vi "ReversedEngineering GetRunTimeMenuTags.vi"(1 "StateMachineCaseSelector":path, 5 "error in":errorcluster) -> (16 "ItemTags":string[](array[string]), 19 "error out":errorcluster)   [LabVIEW 2014]
panel:
  out "data":string
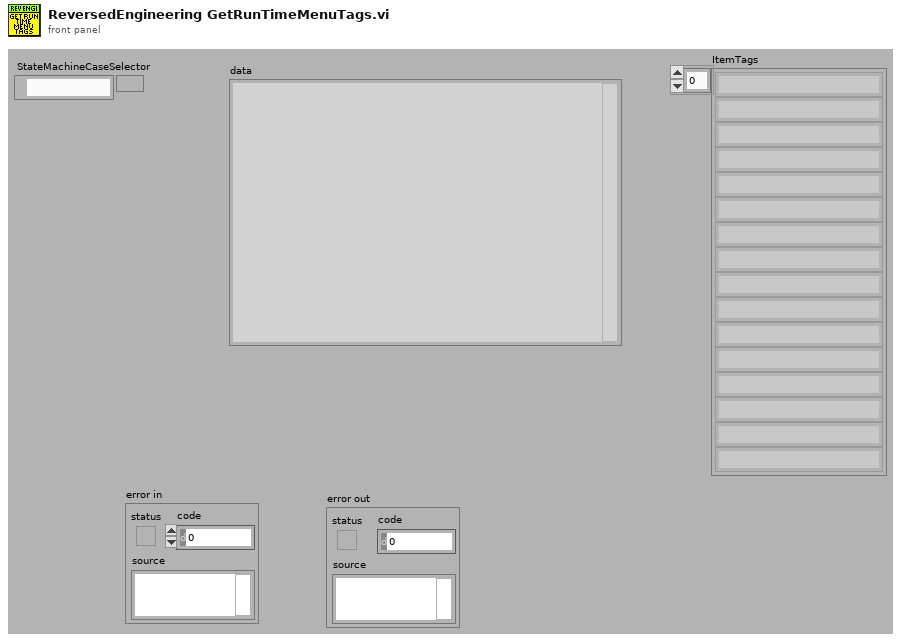
[diagram p1: front panel]
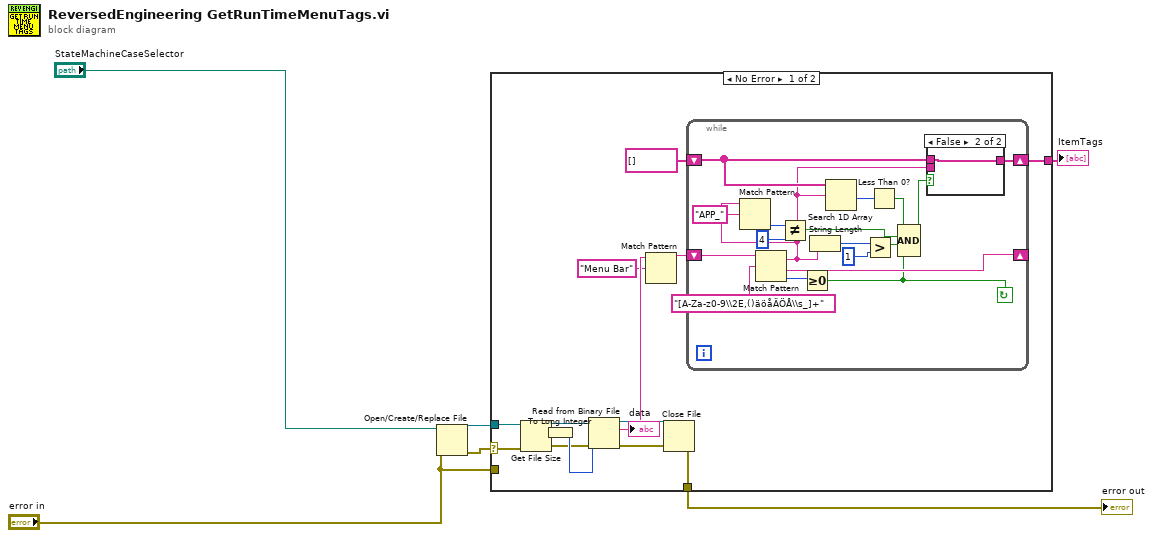
[diagram p0: block diagram]
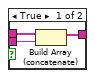
[diagram p2: hidden frame]
diagram:
  n1 = Open/Create/Replace File(file path (use dialog)="StateMachineCaseSelector", error in="error in") -> (refnum out=w6:refnum<file>, error out=w2:errorcluster)  [unwired: 4 in, 1 out]
  n2 = case shown="No Error" w2 {
    selector: w2 -> [w8 _]
    tunnel: w6 -> [w20 _]
    tunnel: [w14 w43] -> w4
    tunnel: [w12 _] -> w3
    tunnel: "error in" -> [_ w43]
    frame No Error {
      n3 = Get File Size(file=w20, error in=w8) -> (refnum out=w17:refnum<file>, size (in bytes)=w7:i64, 0:w18:errorcluster)
      n4 = To Long Integer(number=w7) -> (32bit integer=w19:i32)
      n5 = Read from Binary File(8:w18, 10:w19, 11:w17) -> (0:w15:errorcluster, 2:w11:string, 3:w16:refnum<file>)  [unwired: 4 out]
      "data" <- w11
      n6 = Match Pattern(string=w11, regular expression="Menu Bar") -> (after substring=w10:string)  [unwired: 4 out]
      n7 = Close File(refnum=w16, error in=w15) -> (error out=w14:errorcluster)  [unwired: 1 out]
      n8 = while {
        shift-right: [w36] -> _
        shift-left: w10 -> [w38]
        shift-right: [w35] -> w12
        shift-left: string[] [] -> [w28]
        stop <- w29 continue-if-true
        n9 = Match Pattern(string=w38, regular expression="[A-Za-z0-9\\2E,()äöåÄÖÅ\\s_]+") -> (match substring=w25:string, after substring=w36:string, offset past match=w34:i32)  [unwired: 2 out]
        n10 = Match Pattern(string=w25, regular expression="APP_") -> (offset past match=w23:i32)  [unwired: 4 out]
        n11 = Not Equal?(x=w23, y=4) -> (x != y?=w21:bool)
        n12 = Greater Or Equal To 0?(x=w34) -> (x >= 0?=w29:bool)
        n13 = String Length(string=w25) -> (length=w33:i32)
        n14 = Search 1D Array(1D array=w28, element=w25) -> (index of element=w27:i32)  [unwired: 1 out]
        n15 = Greater?(x=w33, y=1) -> (0:w30:bool)
        n16 = Less Than 0?(x=w27) -> (x < 0?=w26:bool)
        n17 = Compound Arithmetic op=AND(w26, w21, w30, w29) -> (w31:bool)
        n18 = case shown="False" w31 {
          tunnel: w28 -> [w41 w42]
          tunnel: w25 -> [w40 _]
          tunnel: [w39 w42] -> w35
          frame True {
            n19 = Build Array (concatenate)(w41, w40) -> (w39:string[])
          }
          frame False {
          }
        }
      }
    }
    frame Error {
    }
  }
  "error out" <- w4
  "ItemTags" <- w3
